vi "OnDoubleClick2.vi"(0 "XRef":T9, 1 "Point":T7, 2 "Mouse Mods":T5, 3 "State In":T1) -> (14 "Reply":T3, 15 "Fatal Error Out":T2, 16 "State Out":T1)   [LabVIEW 2014, in "TagDB(dev).lvlib" / "tagDB_value.xnode"]
uses:
  tagDB_value.xnode
  <vilib>/XNodeSupport/XNodeXNodeRef.ctl
  <vilib>/XNodeSupport/XNodePoint.ctl
  <vilib>/XNodeSupport/XNodeInt.ctl
  <vilib>/XNodeSupport/XNodeMouseMods.ctl
  <vilib>/XNodeSupport/XNodeBool.ctl
  State.ctl
  <vilib>/XNodeSupport/XNodeStringArray.ctl
  <vilib>/XNodeSupport/XNodeString.ctl
  <vilib>/XNodeSupport/XNodeErrorCluster.ctl
  <vilib>/XNodeSupport/NI_XNodeSupport.lvlib
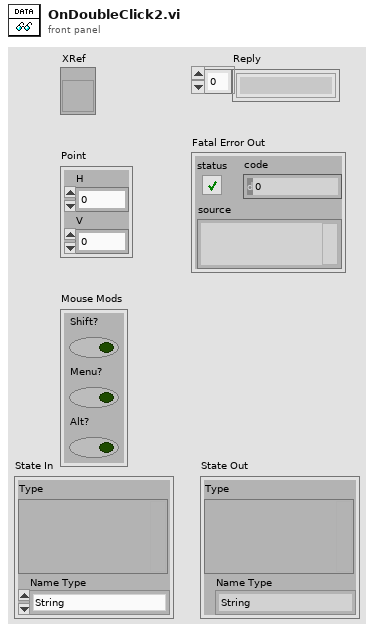
[diagram p1: front panel]
types:
  T1 = typedef "TagDB(dev).lvlib/tagDB_value.xnode/State.ctl" = cluster{"Type":variant, "Name Type":enum16{"String", "RegPattern"}}
  T2 = typedef "NI_XNodeSupport.lvlib/XNodeErrorCluster.ctl" = errorcluster
  T3 = typedef "NI_XNodeSupport.lvlib/XNodeStringArray.ctl" = T4[]
  T4 = typedef "NI_XNodeSupport.lvlib/XNodeString.ctl" = string
  T5 = typedef "NI_XNodeSupport.lvlib/XNodeMouseMods.ctl" = cluster{"Shift?":T6, "Menu?":T6, "Alt?":T6}
  T6 = typedef "NI_XNodeSupport.lvlib/XNodeBool.ctl" = bool
  T7 = typedef "NI_XNodeSupport.lvlib/XNodePoint.ctl" = cluster{"H":T8, "V":T8}
  T8 = typedef "NI_XNodeSupport.lvlib/XNodeInt.ctl" = i32
  T9 = typedef "NI_XNodeSupport.lvlib/XNodeXNodeRef.ctl" = refnum<vi>
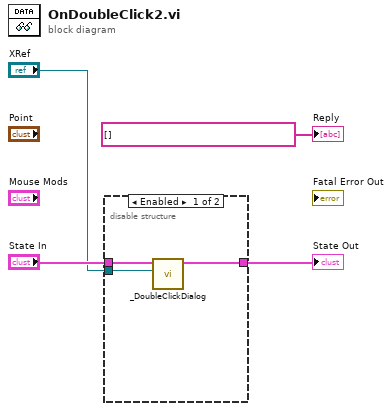
[diagram p0: block diagram]
diagram:
  n1 = disable-structure shown="Enabled" {
    disable-tunnel: "State In" -> [w7 w8]
    disable-tunnel: [w6 w8] -> w3
    disable-tunnel: "XRef" -> [w5 _]
    frame Enabled {
      n2 = call "_DoubleClickDialog.vi"("XRef"=w5, "State In"=w7) -> ("State Out"=w6:T1)  [unwired: 8 in, 1 out]
    }
    frame Disabled {
    }
  }
  "State Out" <- w3
  "Reply" <- T3 [] ("Reply")
